vi "SCE_flatten_pixmap.vi"(6 "colors":u32[](array[numeric]), 7 "top left":cluster{"x":i16, "y":i16}, 10 "8-bit pixmap":u8[][](array[numeric])) -> (2 "image data":T1)   [LabVIEW 2018]
doc: "Converts pixmap data from a 2D array to a 1D array."
uses:
  <vilib>/picture/picture.llb/imagedata.ctl
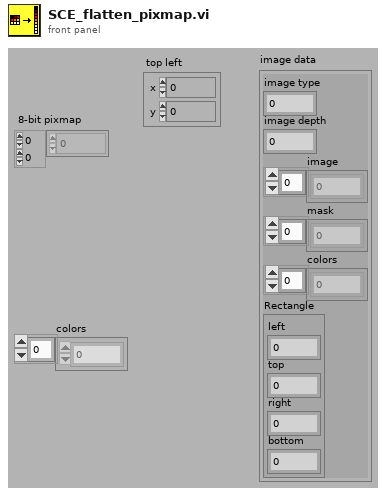
[diagram p1: front panel]
types:
  T1 = typedef "imagedata.ctl" = cluster{"image type":i32, "image depth":i32, "image":u8[], "mask":u8[], "colors":u32[], "Rectangle":cluster{"left":i16, "top":i16, "right":i16, "bottom":i16}}
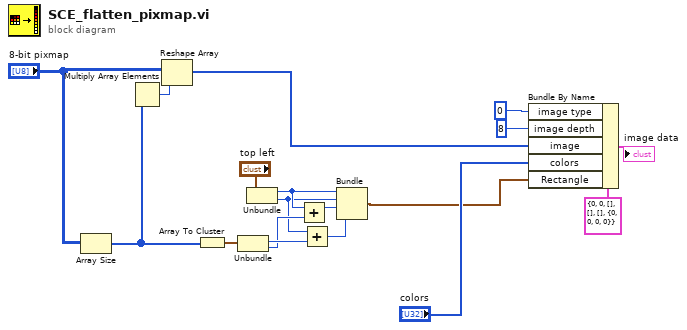
[diagram p0: block diagram]
diagram:
  n1 = Array Size(array="8-bit pixmap") -> (size(s)=w1:i32[])
  n2 = Multiply Array Elements(1:w1) -> (0:w2:i32)
  n3 = Reshape Array("8-bit pixmap", w2) -> (w3:u8[])
  n4 = Array To Cluster(array=w1) -> (cluster=w17:cluster{"[0]":i32, "[1]":i32})
  n5 = Unbundle(w17) -> ("[0]"=w16:i32, "[1]"=w13:i32)
  n6 = Unbundle("top left") -> ("x"=w14:i16, "y"=w12:i16)
  n7 = Add(x=w14, y=w13) -> (x+y=w10:i32)
  n8 = Add(x=w12, y=w16) -> (x+y=w11:i32)
  n9 = Bundle("x"=w14, "y"=w12, w10, w11) -> (w5:cluster{"x":i16, "y":i16, i32, i32})  [unwired: 1 in]
  n10 = Bundle By Name(cluster=T1 {"image type"=0, "image depth"=0, "image"=[], "mask"=[], "colors"=[], "Rectangle"={"left"=0, "top"=0, "right"=0, "bottom"=0}} ("image data"), "image type"=u16 0, "image depth"=8, "image"=w3, "colors"="colors", "Rectangle"=w5) -> (→"image data":T1)
